vi "Get_File_Info_Listing.vi"(0 "path":path) -> (1 "Path":path[](array[path]), 2 "Last Mod":dbl[](array[numeric]), 3 "Size":i64[](array[numeric]))   [LabVIEW 2011]
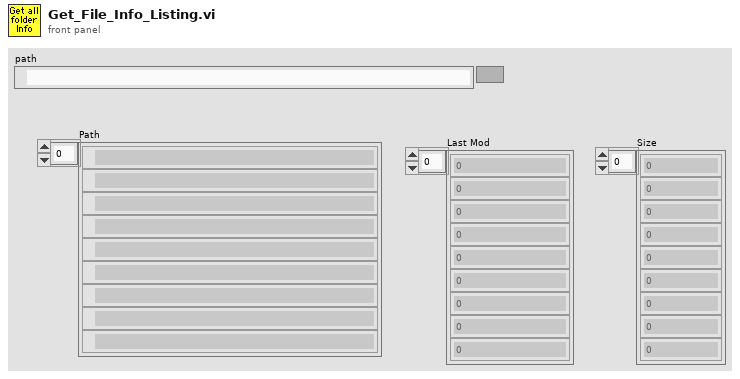
[diagram p1: front panel]
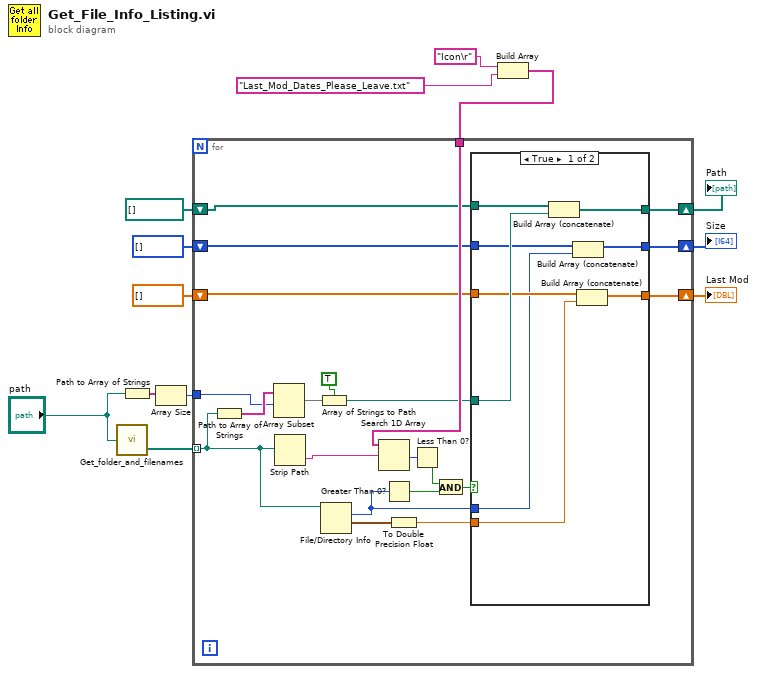
[diagram p0: block diagram]
diagram:
  n1 = call "Get_folder_and_filenames.vi"("file path (dialog if empty)"="path") -> ("Files"=w9:path[])  [unwired: 1 out]
  n2 = Path to Array of Strings(0:"path") -> (2:w10:string[])  [unwired: 1 out]
  n3 = Array Size(array=w10) -> (size(s)=w11:i32)
  n4 = Build Array("Icon\r", "Last_Mod_Dates_Please_Leave.txt" ("name or relative path")) -> (w13:string[])
  n5 = for {
    tunnel: w9 -> [w20] mode=indexing
    tunnel: w11 -> [w33]
    shift-right: [w25] -> w3
    shift-left: path[] [] -> [w27]
    tunnel: w13 -> [w31]
    shift-right: [w23] -> w4
    shift-left: i64[] [] -> [w24]
    shift-right: [w21] -> w5
    shift-left: dbl[] [] -> [w22]
    n6 = Path to Array of Strings(0:w20) -> (2:w34:string[])  [unwired: 1 out]
    n7 = Array Subset(array=w34, index=w33) -> (w29:string[])  [unwired: 1 in]
    n8 = Strip Path(path=w20) -> (name=w32:string)  [unwired: 1 out]
    n9 = Array of Strings to Path(0:w29, 1:TRUE ("relative")) -> (2:w26:path)
    n10 = File/Directory Info(path=w20) -> (size=w16:i64, last mod=w15:timestamp)  [unwired: 1 in, 5 out]
    n11 = Search 1D Array(1D array=w31, element=w32) -> (index of element=w30:i32)  [unwired: 1 out]
    n12 = Greater Than 0?(x=w16) -> (x > 0?=w18:bool)
    n13 = To Double Precision Float(number=w15) -> (double precision float=w14:dbl)
    n14 = Less Than 0?(x=w30) -> (x < 0?=w19:bool)
    n15 = And(x=w19, y=w18) -> (x .and. y?=w17:bool)
    n16 = case shown="True" w17 {
      tunnel: w27 -> [w43 w46]
      tunnel: w26 -> [w42 _]
      tunnel: [w41 w46] -> w25
      tunnel: w24 -> [w40 w45]
      tunnel: [w39 w45] -> w23
      tunnel: w22 -> [w38 w44]
      tunnel: [w37 w44] -> w21
      tunnel: w14 -> [w36 _]
      tunnel: w16 -> [w35 _]
      frame True {
        n17 = Build Array (concatenate)(w43, w42) -> (w41:path[])
        n18 = Build Array (concatenate)(w40, w35) -> (w39:i64[])
        n19 = Build Array (concatenate)(w38, w36) -> (w37:dbl[])
      }
      frame False {
      }
    }
  }
  "Last Mod" <- w5
  "Size" <- w4
  "Path" <- w3
